vi "OnDeviceListChangedCallback.vi"(4 "Device List Change":refnum<vi>, 6 "Control Ref":refnum<k7>, 7 "Event Common Data":T1) -> ()   [LabVIEW 2016]
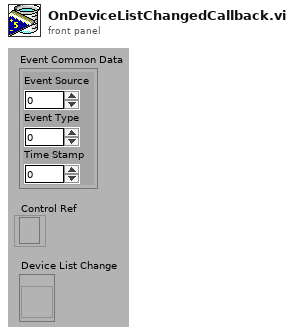
[diagram p1: front panel]
types:
  T1 = cluster{"Event Source":i32, "Event Type":u32, "Time Stamp":u32}
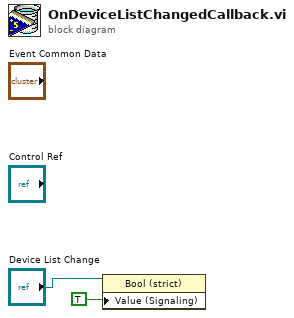
[diagram p0: block diagram]
diagram:
  n1 = property class="Bool (strict)"(reference="Device List Change", "Value (Signaling)"=TRUE ("Value")) -> ()  [unwired: 1 in, 2 out]
